vi "addyaxis.vi"(1 "y axis labels":dbl[](array[numeric]), 3 "input array":dbl[][](array[numeric])) -> (0 "Array":dbl[][](array[numeric]))   [LabVIEW 2013]
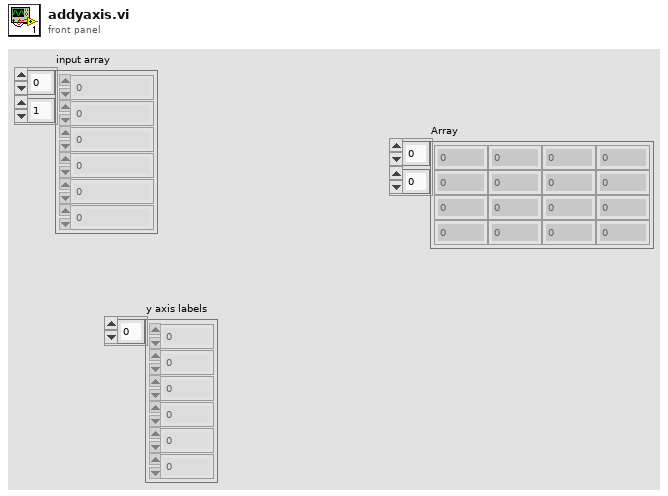
[diagram p1: front panel]
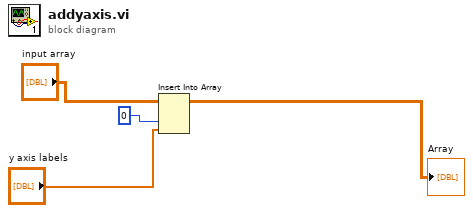
[diagram p0: block diagram]
diagram:
  n1 = Insert Into Array(array="input array", index (col)=0, new element="y axis labels") -> (→"Array":dbl[][])  [unwired: 1 in]
